vi "deluxe.vi"(4 "Current cycle switch":refnum<vi>, 6 "timer":refnum<vi>, 7 "Next state in":T1, 9 "Stop":refnum<vi>, 10 "Vehicle out of position":refnum<vi>, 11 "Current cycle indicator":refnum<vi>) -> (2 "stop":bool, 3 "Next state out":T1)   [LabVIEW 2024]
uses:
  purchase_selection_state1.ctl
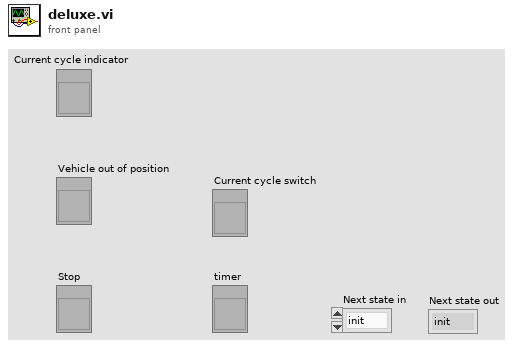
[diagram p1: front panel]
types:
  T1 = typedef "purchase_selection_state1.ctl" = enum16{"init", "wait", "underbody wash", "main wash", "air dry", "log", "end"}
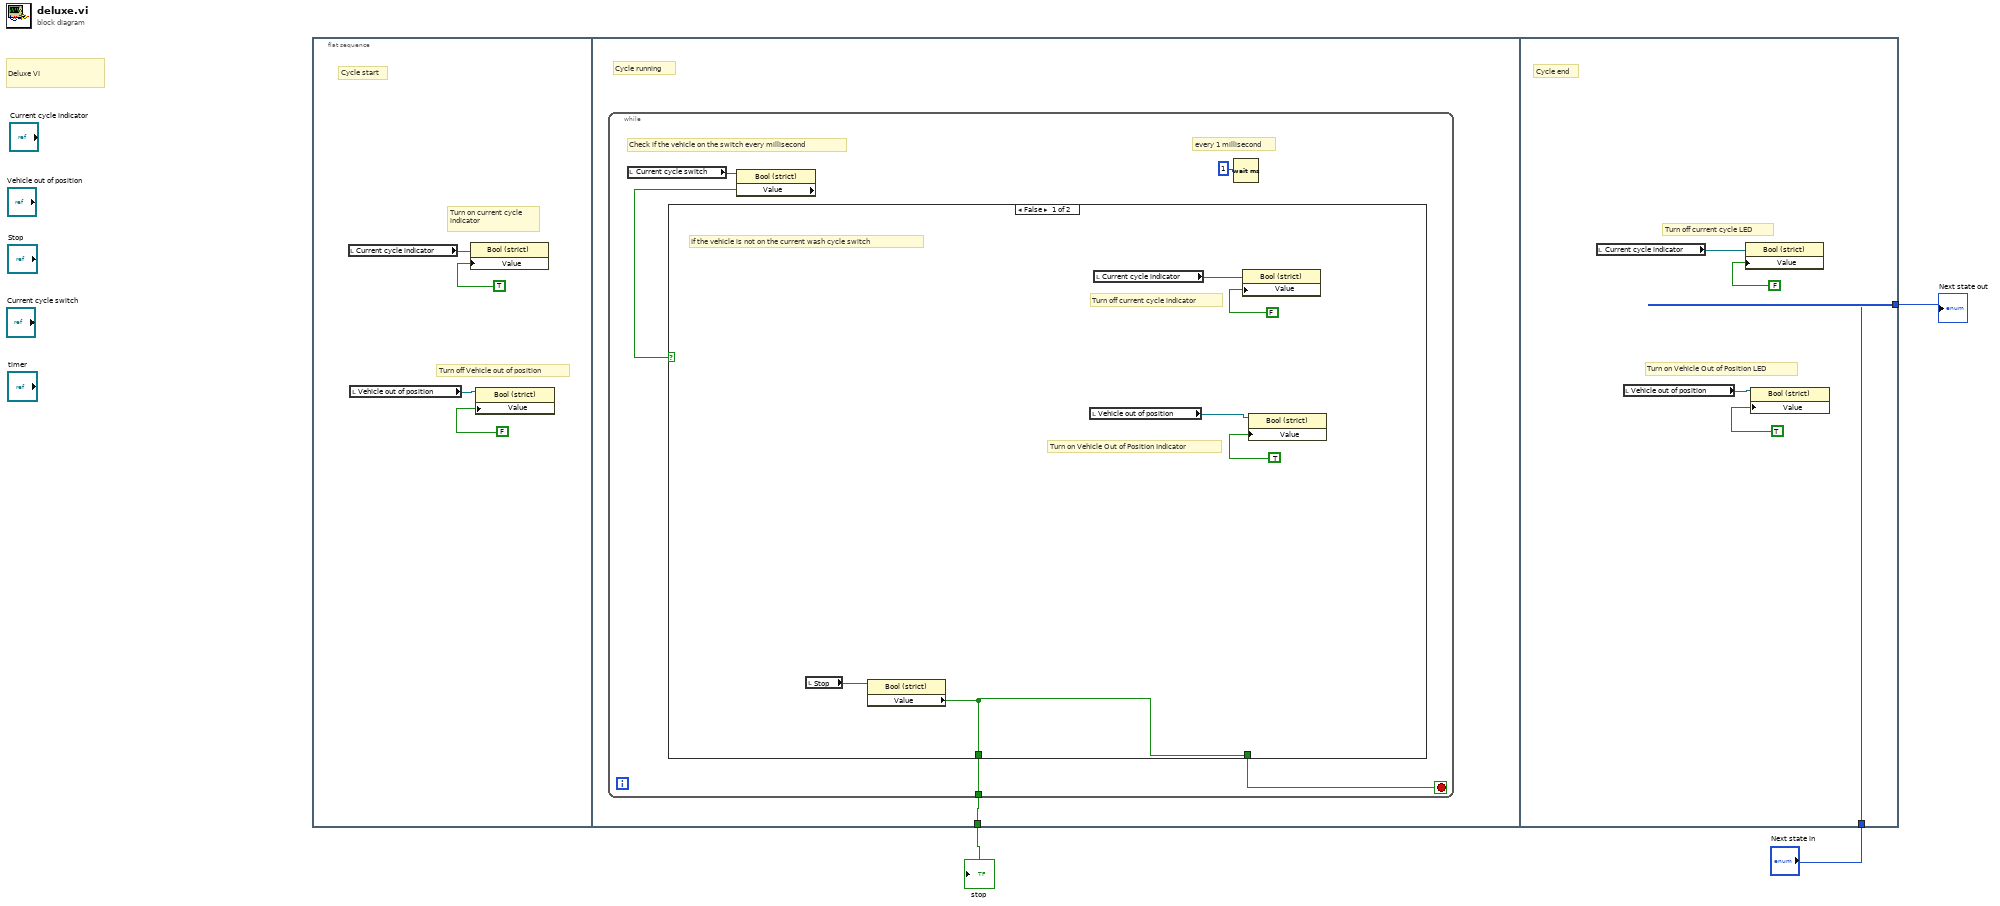
[diagram p0: block diagram]
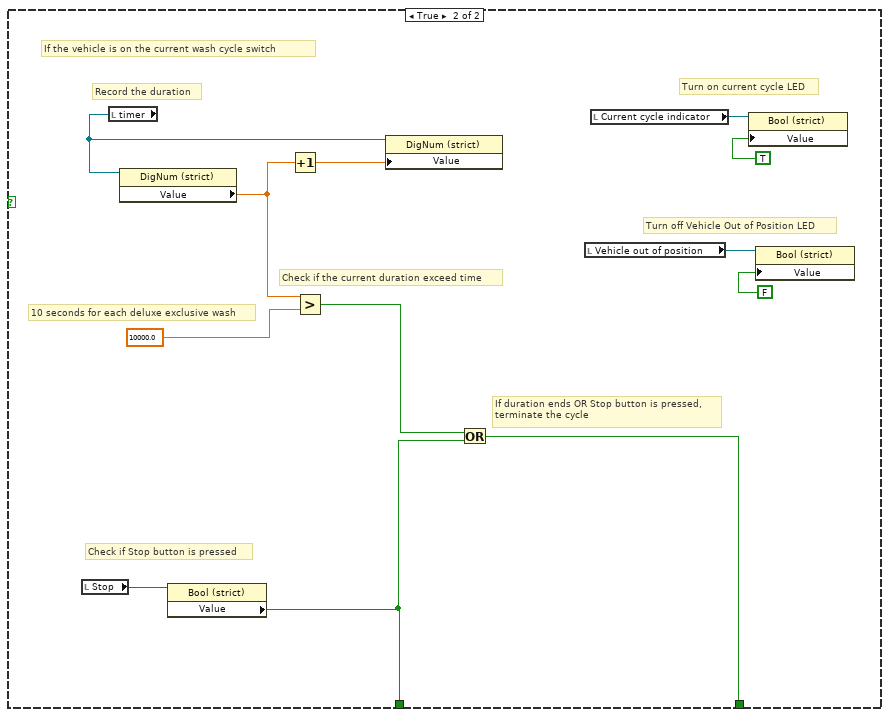
[diagram p2: hidden frame]
diagram:
  # "Deluxe VI"
  n1 = flat-sequence {
    tunnel: [w8] -> w1
    tunnel: "Next state in" -> [w36]
    tunnel: [w36] -> w3
    frame #0 {
      # "Cycle start"
      # "Turn off Vehicle out of position"
      # "Turn on current cycle\nindicator"
      n2 = local read "Current cycle indicator"() -> (w4:refnum<vi>)
      n3 = local read "Vehicle out of position"() -> (w5:refnum<vi>)
      n4 = property class="Bool (strict)"(reference=w4, "Value"=TRUE ("Under Body Wash")) -> ()  [unwired: 1 in, 2 out]
      n5 = property class="Bool (strict)"(reference=w5, "Value"=FALSE ("Under Body Wash")) -> ()  [unwired: 1 in, 2 out]
    }
    frame #1 {
      # "Cycle running"
      n6 = while {
        tunnel: [w11] -> w8
        stop <- w12 stop-if-true
        # "every 1 millisecond"
        # "Check if the vehicle on the switch every millisecond"
        n7 = local read "Current cycle switch"() -> (w10:refnum<vi>)
        n8 = property class="Bool (strict)"(reference=w10) -> ("Value"=w9:bool)  [unwired: 1 in, 2 out]
        n9 = case shown="False" w9 {
          tunnel: [w19 w20] -> w12
          tunnel: [w19 w27] -> w11
          frame False {
            # "Turn on Vehicle Out of Position Indicator"
            # "Turn off current cycle indicator"
            # "If the vehicle is not on the current wash cycle switch"
            n10 = local read "Stop"() -> (w14:refnum<vi>)
            n11 = property class="Bool (strict)"(reference=w14) -> ("Value"=w19:bool)  [unwired: 1 in, 2 out]
            n12 = local read "Vehicle out of position"() -> (w16:refnum<vi>)
            n13 = local read "Current cycle indicator"() -> (w15:refnum<vi>)
            n14 = property class="Bool (strict)"(reference=w15, "Value"=FALSE ("Under Body Wash")) -> ()  [unwired: 1 in, 2 out]
            n15 = property class="Bool (strict)"(reference=w16, "Value"=TRUE ("Under Body Wash")) -> ()  [unwired: 1 in, 2 out]
          }
          frame True {
            # "Turn off Vehicle Out of Position LED"
            # "Turn on current cycle LED"
            # "If duration ends OR Stop button is pressed,\nterminate the cycle"
            # "Check if Stop button is pressed"
            # "Check if the current duration exceed time"
            # "10 seconds for each deluxe exclusive wash"
            # "Record the duration"
            # "If the vehicle is on the current wash cycle switch"
            n16 = local read "Stop"() -> (w22:refnum<vi>)
            n17 = local read "timer"() -> (w21:refnum<vi>)
            n18 = property class="DigNum (strict)"(reference=w21) -> ("Value"=w30:dbl)  [unwired: 1 in, 2 out]
            n19 = property class="Bool (strict)"(reference=w22) -> ("Value"=w27:bool)  [unwired: 1 in, 2 out]
            n20 = Increment(x=w30) -> (x+1=w31:dbl)
            n21 = Greater?(x=w30, y=10000.0) -> (0:w28:bool)
            n22 = property class="DigNum (strict)"(reference=w21, "Value"=w31) -> ()  [unwired: 1 in, 2 out]
            n23 = Or(x=w28, y=w27) -> (x .or. y?=w20:bool)
            n24 = local read "Vehicle out of position"() -> (w25:refnum<vi>)
            n25 = local read "Current cycle indicator"() -> (w26:refnum<vi>)
            n26 = property class="Bool (strict)"(reference=w26, "Value"=TRUE ("Under Body Wash")) -> ()  [unwired: 1 in, 2 out]
            n27 = property class="Bool (strict)"(reference=w25, "Value"=FALSE ("Under Body Wash")) -> ()  [unwired: 1 in, 2 out]
          }
        }
        n28 = Wait (ms)(milliseconds to wait=u32 1) -> ()  [unwired: 1 out]
      }
    }
    frame #2 {
      # "Turn on Vehicle Out of Position LED"
      # "Turn off current cycle LED"
      # "Cycle end"
      n29 = local read "Current cycle indicator"() -> (w35:refnum<vi>)
      n30 = local read "Vehicle out of position"() -> (w34:refnum<vi>)
      n31 = property class="Bool (strict)"(reference=w35, "Value"=FALSE ("Under Body Wash")) -> ()  [unwired: 1 in, 2 out]
      n32 = property class="Bool (strict)"(reference=w34, "Value"=TRUE ("Under Body Wash")) -> ()  [unwired: 1 in, 2 out]
    }
  }
  "Next state out" <- w3
  "stop" <- w1
